vi "Rig Config - Load Filenames.vi"(8 "Error IN":errorcluster) -> (0 "Error OUT":errorcluster, 3 "Rig Config File Names OUT":string[](array[string]))   [LabVIEW 2018]
uses:
  Globals/Global - Configuration Options.vi
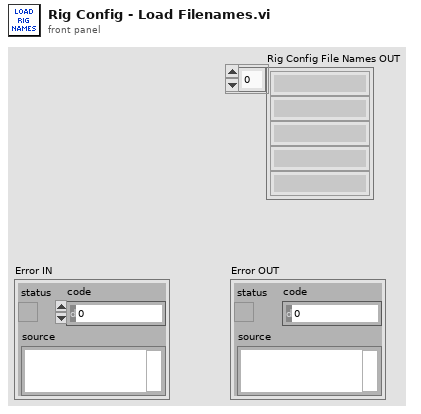
[diagram p1: front panel]
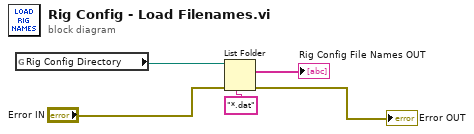
[diagram p0: block diagram]
diagram:
  n1 = global read "Global - Configuration Options.vi" "Rig Config Directory"() -> (w1:path)
  n2 = List Folder(path=w1, pattern="*.dat", error in="Error IN") -> (filenames=→"Rig Config File Names OUT":string[], error out=→"Error OUT":errorcluster)  [unwired: 1 in, 2 out]
